vi "Receive Value Change Event.vi"(8 "error in (no error)":errorcluster, 10 "ValueChangeMsg":refnum<class "ValueChangeMsg.lvclass">, 11 "For Loop Dialog In":refnum<class "For Loop Dialog.lvclass">) -> (0 "error out":errorcluster, 3 "For Loop Dialog Out":refnum<class "For Loop Dialog.lvclass">)   [LabVIEW 2017, in "For Loop Dialog.lvclass"]
doc: "<License>\nCopyright © 2017 Composed Systems, LLC | All rights reserved\nwww.composed.io\n\nAuthor: Ethan Stern <ethan.stern@composed.io>\n\nThis software is provided \"AS IS\" WITHOUT WARRANTIES, either express or implied, AND IS FOR EDUCATIONAL PURPOSES ONLY.\n</License>"
uses:
  For Loop Dialog.lvclass
  ITest Executive Builder Dialog/ITest Executive Builder Dialog.lvclass
  <vilib>/gpm_packages/@cs/mva-viewable/Source/ActorEvents/IEventAggregator Messages/ValueChangeMsg/ValueChangeMsg.lvclass
  <vilib>/ActorFramework/Actor/Actor.lvclass
  <vilib>/ActorFramework/Stop Msg/Stop Msg.lvclass
  C:/Program Files (x86)/National Instruments/LabVIEW 2017/vi.lib/ActorFramework/Actor/Actor.lvclass
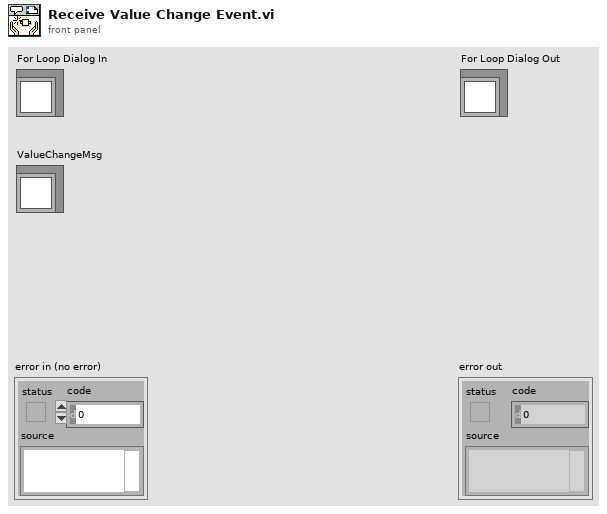
[diagram p1: front panel]
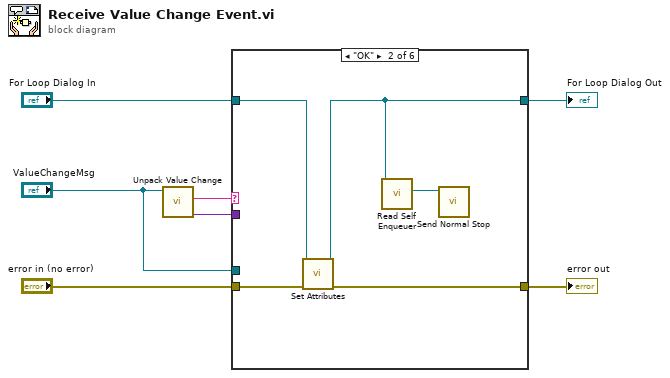
[diagram p0: block diagram]
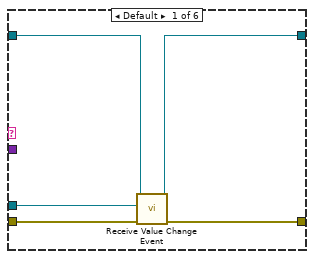
[diagram p2: hidden frame]
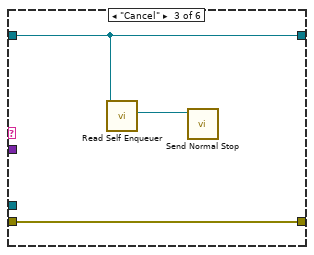
[diagram p3: hidden frame]
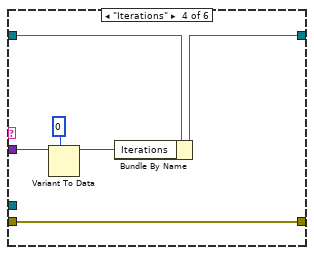
[diagram p4: hidden frame]
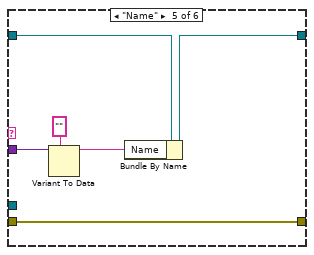
[diagram p5: hidden frame]
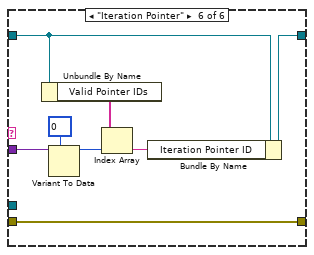
[diagram p6: hidden frame]
diagram:
  n1 = call <vilib>:"Unpack Value Change.vi"("ValueChangeMsg"="ValueChangeMsg") -> ("New Value"=w1:variant, "Control Label"=w2:string)  [unwired: 6 in, 3 out]
  n2 = case shown="\"OK\"" w2 {
    tunnel: [w12 w15 w20 w26 w32 w40] -> w7
    tunnel: [w11 w14 w19 w21 w27 w38] -> w6
    tunnel: "error in (no error)" -> [w10 w16 w20 w26 w32 w40]
    tunnel: "For Loop Dialog In" -> [w9 w13 w19 w22 w28 w36]
    tunnel: "ValueChangeMsg" -> [w8 _ _ _ _ _]
    tunnel: w1 -> [_ _ _ w25 w31 w39]
    frame Default {
      n3 = call-parent "Receive Value Change Event.vi"("error in (no error)"=w10, "ValueChangeMsg"=w8, "IViewable In"=w9) -> ("error out"=w12:errorcluster, "IViewable Out"=w11:refnum<class "For Loop Dialog.lvclass">)  [unwired: 7 in]
    }
    frame "OK" {
      n4 = call-dynamic "Set Attributes.vi"("error in (no error)"=w16, "For Loop Dialog in"=w13) -> ("error out"=w15:errorcluster, "For Loop Dialog out"=w14:refnum<class "For Loop Dialog.lvclass">)  [unwired: 8 in]
      n5 = call <vilib>:"Read Self Enqueuer.vi"("Actor"=w14) -> ("Self Enqueuer"=w17:refnum<class "Message Enqueuer.lvclass">)  [unwired: 10 in]
      n6 = call <vilib>:"Send Normal Stop.vi"("Message Enqueuer"=w17) -> ()  [unwired: 10 in, 1 out]
    }
    frame "Cancel" {
      n7 = call <vilib>:"Read Self Enqueuer.vi"("Actor"=w19) -> ("Self Enqueuer"=w18:refnum<class "Message Enqueuer.lvclass">)  [unwired: 10 in]
      n8 = call <vilib>:"Send Normal Stop.vi"("Message Enqueuer"=w18) -> ()  [unwired: 10 in, 1 out]
    }
    frame "Iterations" {
      n9 = Variant To Data(type=u32 0 ("Iterations"), Variant=w25) -> (data=w23:u32)  [unwired: 1 in, 1 out]
      n10 = Bundle By Name(cluster=w22, "Iterations"=w23) -> (w21:refnum<class "For Loop Dialog.lvclass">)
    }
    frame "Name" {
      n11 = Variant To Data(type="" ("Iterations"), Variant=w31) -> (data=w29:string)  [unwired: 1 in, 1 out]
      n12 = Bundle By Name(cluster=w28, "Name"=w29) -> (w27:refnum<class "For Loop Dialog.lvclass">)
    }
    frame "Iteration Pointer" {
      w37 = u16 0 items=[""] ("Iteration Pointer")
      n13 = Unbundle By Name(w36) -> ("Valid Pointer IDs"=w34:string[])
      n14 = Variant To Data(type=w37, Variant=w39) -> (data=w35:u16)  [unwired: 1 in, 1 out]
      n15 = Index Array(array=w34, index=w35) -> (element=w33:string)
      n16 = Bundle By Name(cluster=w36, "Iteration Pointer ID"=w33) -> (w38:refnum<class "For Loop Dialog.lvclass">)
    }
  }
  "error out" <- w7
  "For Loop Dialog Out" <- w6
